vi "programControlNotifier.vi"(8 "error in (no error)":errorcluster, 10 "Message in":T1, 11 "Enum":T2) -> (0 "error out":errorcluster, 2 "message out":T1)   [LabVIEW 2017, in "programControl.lvlib"]
uses:
  programControl.lvlib
  TypeDefs/notifierFGVStates.ctl
  TypeDefs/notificationMessage.ctl
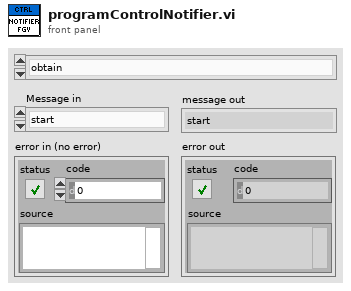
[diagram p1: front panel]
types:
  T1 = typedef "programControl.lvlib/notificationMessage.ctl" = enum16{"start", "wait", "run", "end"}
  T2 = typedef "programControl.lvlib/notifierFGVStates.ctl" = enum16{"obtain", "send", "wait for notification", "release"}
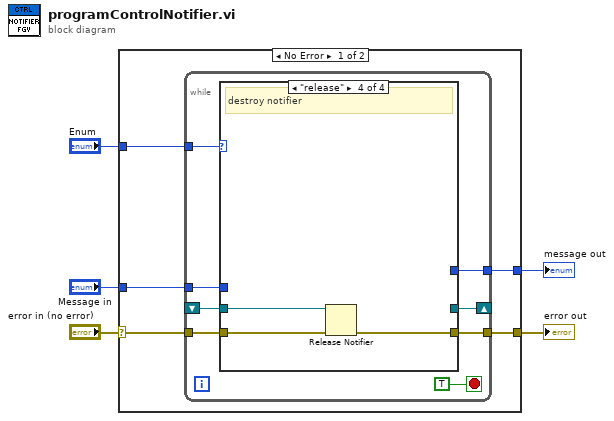
[diagram p0: block diagram]
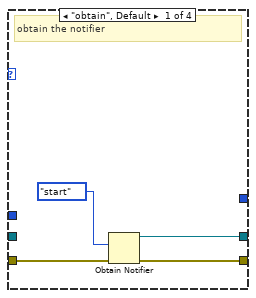
[diagram p2: hidden frame]
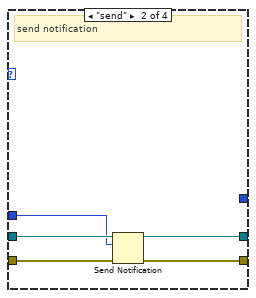
[diagram p3: hidden frame]
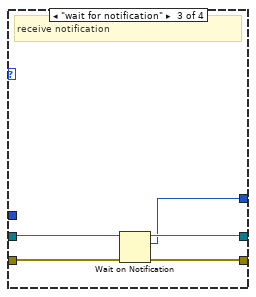
[diagram p4: hidden frame]
diagram:
  n1 = case shown="No Error" "error in (no error)" {
    selector: "error in (no error)" -> [w9 w36]
    tunnel: [w8 w36] -> w4
    tunnel: "Enum" -> [w10 _]
    tunnel: "Message in" -> [w7 _]
    tunnel: [w6 _] -> w1
    frame No Error {
      n2 = while {
        tunnel: w10 -> [w17]
        tunnel: w9 -> [w16]
        tunnel: [w15] -> w8
        shift-right: [w14] -> _
        shift-left: _ -> [w13]
        tunnel: w7 -> [w12]
        tunnel: [w11] -> w6
        stop <- TRUE stop-if-true
        n3 = case shown="\"release\"" w17 {
          tunnel: w16 -> [w22 w27 w32 w34]
          tunnel: [w21 w26 w31 w33] -> w15
          tunnel: [w20 w25 w30 _] -> w14
          tunnel: w13 -> [_ w24 w29 w35]
          tunnel: w12 -> [_ w23 _ _]
          tunnel: [_ _ w28 _] -> w11
          frame "obtain", Default {
            # "obtain the notifier"
            n4 = Obtain Notifier(notification data type=notificationMessage."start", error in (no error)=w22) -> (notifier out=w20:refnum<notifier>, error out=w21:errorcluster)  [unwired: 2 in, 1 out]
          }
          frame "send" {
            # "send notification"
            n5 = Send Notification(notification=w23, notifier=w24, error in (no error)=w27) -> (notifier out=w25:refnum<notifier>, error out=w26:errorcluster)
          }
          frame "wait for notification" {
            # "receive notification"
            n6 = Wait on Notification(notifier=w29, error in (no error)=w32) -> (notifier out=w30:refnum<notifier>, notification=w28:T1, error out=w31:errorcluster)  [unwired: 2 in, 1 out]
          }
          frame "release" {
            # "destroy notifier"
            n7 = Release Notifier(notifier=w35, error in (no error)=w34) -> (error out=w33:errorcluster)  [unwired: 1 in, 2 out]
          }
        }
      }
    }
    frame Error {
    }
  }
  "error out" <- w4
  "message out" <- w1
